vi "ChangeAmpWFG.vi"(0 "object in":refnum<class "AD2andExtAWG.lvclass">, 2 "AmplitudeCh1&2":T1, 5 "error in (no error)":errorcluster) -> (14 "object out":refnum<class "AD2andExtAWG.lvclass">, 19 "error out":errorcluster)   [LabVIEW 2023, in "AD2andExtAWG.lvclass"]
uses:
  AD2andExtAWG.lvclass
  AD2andExtAWG.lvclass/AD2andExtAWG.ctl
  AFG3022B_class/AFG3022B.lvclass
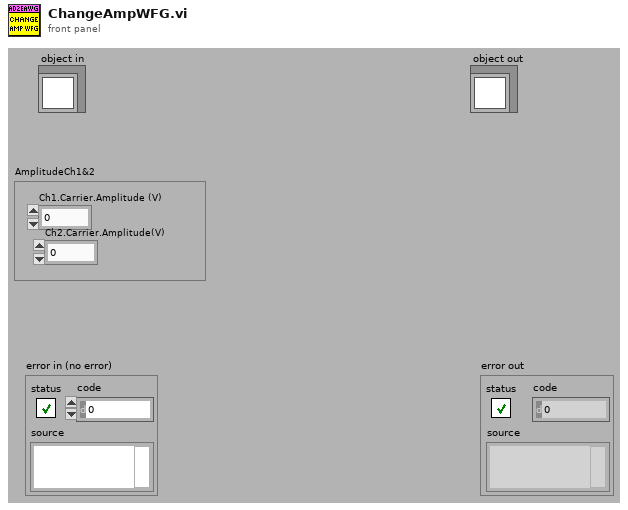
[diagram p1: front panel]
types:
  T1 = cluster{"Ch1.Carrier.Amplitude (V)":dbl, "Ch2.Carrier.Amplitude(V)":dbl}
  T2 = cluster{"ConfigDataCh1":cluster{"Frequency Hz (1000 Hz)":dbl, "Waveform Function (0: Sine)":u16, "Amplitude (1 Vpp)":dbl, "DC Offset (0.00 V)":dbl, "Phase Level (-1)":dbl, "Phase Unit (0: Radian)":u16}, "ConfigDataCh2":cluster{"Frequency Hz (1000 Hz)":dbl, "Waveform Function (0: Sine)":u16, "Amplitude (1 Vpp)":dbl, "DC Offset (0.00 V)":dbl, "Phase Level (-1)":dbl, "Phase Unit (0: Radian)":u16}}
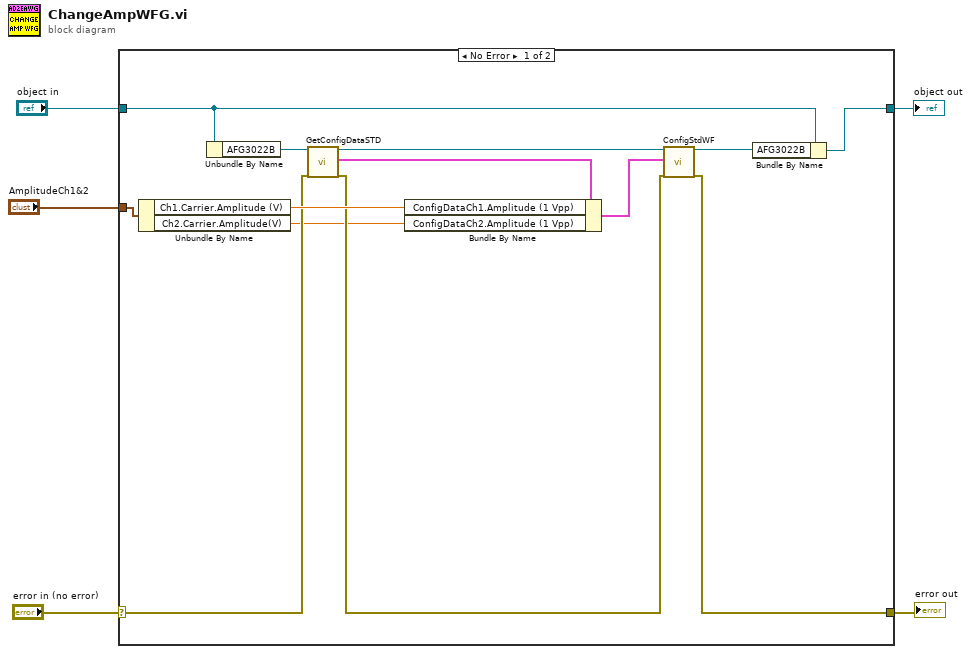
[diagram p0: block diagram]
diagram:
  n1 = case shown="No Error" "error in (no error)" {
    selector: "error in (no error)" -> [w14 w20]
    tunnel: [w12 w20] -> w4
    tunnel: [w11 w19] -> w2
    tunnel: "object in" -> [w10 w19]
    tunnel: "AmplitudeCh1&2" -> [w16 _]
    frame No Error {
      n2 = Unbundle By Name(w16) -> ("Ch1.Carrier.Amplitude (V)"=w15:dbl, "Ch2.Carrier.Amplitude(V)"=w7:dbl)
      n3 = Unbundle By Name(w10) -> ("AFG3022B"=w18:refnum<class "AFG3022B.lvclass">)
      n4 = call-dynamic "GetConfigDataSTD.vi"("object in"=w18, "error in (no error)"=w14) -> ("object out"=w17:refnum<class "AFG3022B.lvclass">, "Configdatastd"=w8:T2, "error out"=w13:errorcluster)  [unwired: 15 in]
      n5 = Bundle By Name(cluster=w8, "ConfigDataCh1.Amplitude (1 Vpp)"=w15, "ConfigDataCh2.Amplitude (1 Vpp)"=w7) -> (w6:T2)
      n6 = call-dynamic "ConfigStdWF.vi"("object in"=w17, "Configdatastd"=w6, "error in (no error)"=w13) -> ("object out"=w9:refnum<class "AFG3022B.lvclass">, "error out"=w12:errorcluster)  [unwired: 15 in]
      n7 = Bundle By Name(cluster=w10, "AFG3022B"=w9) -> (w11:refnum<class "AD2andExtAWG.lvclass">)
    }
    frame Error {
    }
  }
  "error out" <- w4
  "object out" <- w2
